vi "Draw Goal.vi"(7 "Grid Size (10)":i32=10, 11 "Position":T1) -> (3 "Picture":picture)   [LabVIEW 2020, in "App.lvlib" / "MazeUI.lvclass"]
uses:
  MazeUI.lvclass
  Maze/Position.ctl
  Maze/Maze.lvlib
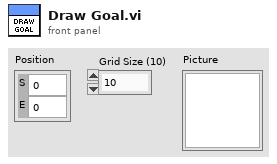
[diagram p1: front panel]
types:
  T1 = typedef "Maze.lvlib/Position.ctl" = cluster{"S":i32, "E":i32}
  T2 = cluster{"Width":u16, "Style":enum32{"Solid", "Dash", "Dot", "DashDot", "DashDotDot"}}
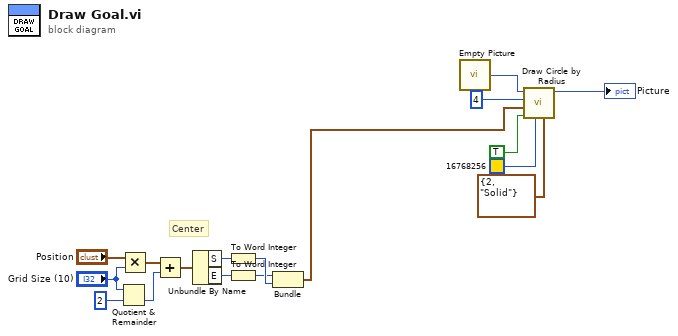
[diagram p0: block diagram]
diagram:
  # "Center"
  n1 = Quotient & Remainder(x="Grid Size (10)", y=2) -> (floor(x/y)=w13:i32)  [unwired: 1 out]
  n2 = Multiply(x="Position", y="Grid Size (10)") -> (x*y=w14:T1)
  n3 = Add(x=w14, y=w13) -> (x+y=w12:T1)
  n4 = Unbundle By Name(w12) -> ("S"=w10:i32, "E"=w11:i32)
  n5 = To Word Integer(number=w10) -> (16bit integer=w9:i16)
  n6 = To Word Integer(number=w11) -> (16bit integer=w8:i16)
  n7 = Bundle(w8, w9) -> (w1:cluster{i16, i16})  [unwired: 1 in]
  n8 = call "Empty Picture"() -> ("empty picture"=w7:picture)
  n9 = call <vilib>:"Draw Circle by Radius.vi"("pen"=T2 {"Width"=2, "Style"=enum."Solid"}, "color(black)"=u32 16768256, "fill?(F)"=TRUE, "pixel center"=w1, "radius"=i16 4, "picture"=w7) -> ("new picture"=→"Picture":picture)  [unwired: 5 in]
